vi "breaking_vigenere.vi"() -> ()   [LabVIEW 2021]
panel:
  in  "OK Button":bool
  in  "KEY":string
  out "Key Lenght":u8
  in  "freq":dbl
  out "Key":string
  out "Testo in chiaro":string
  in  "decifra":bool
  in  "Testo cifrato":string
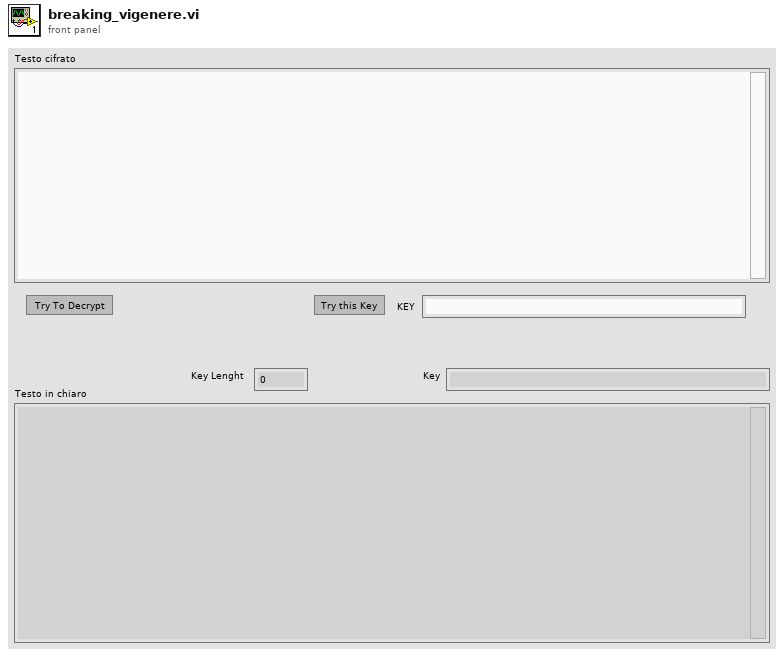
[diagram p1: front panel]
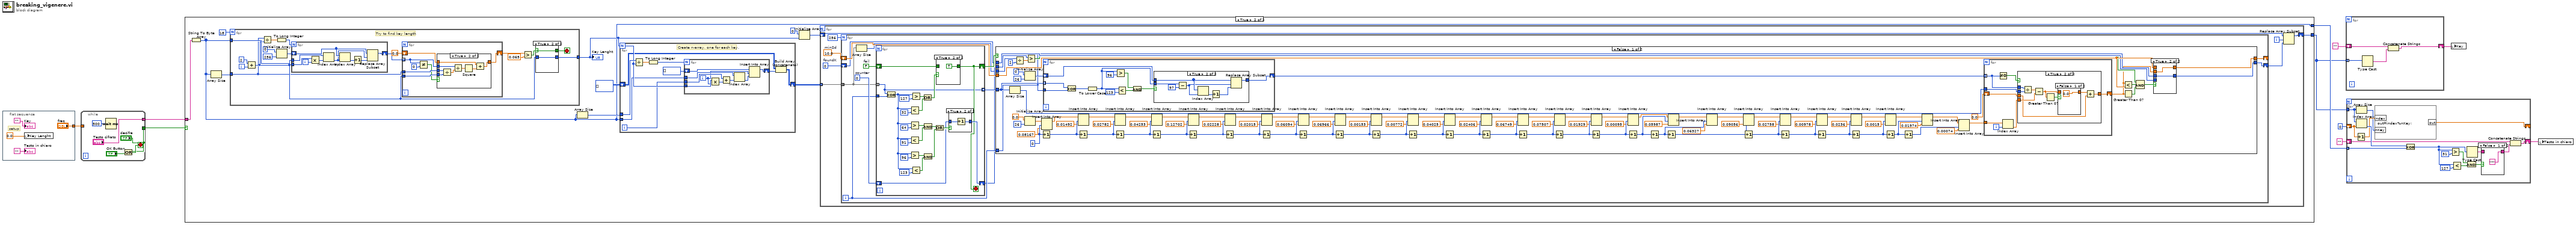
[diagram p0: block diagram]
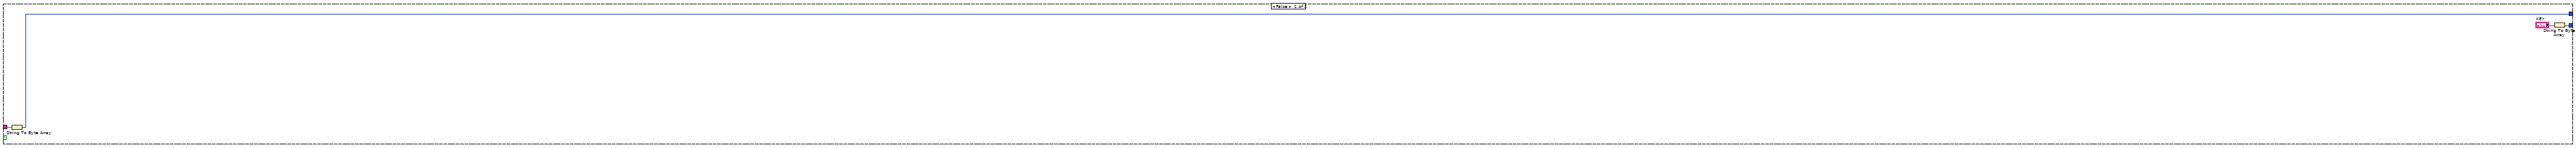
[diagram p2: hidden frame]
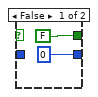
[diagram p3: hidden frame]
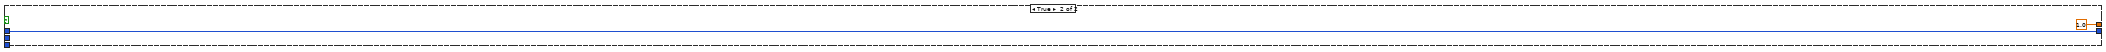
[diagram p9: hidden frame]
diagram:
  n1 = flat-sequence {
    tunnel: ["freq"] -> w5
    frame #0 {
      # "setup"
      n2 = local write "Key Lenght"(0.0 ("Key Lenght")) -> ()
      "Key" <- ""
      "Testo in chiaro" <- ""
    }
  }
  n3 = while {
    tunnel: ["Testo cifrato"] -> w10
    tunnel: w5 -> [_]
    tunnel: ["decifra"] -> w4
    stop <- w16 stop-if-true
    n4 = Wait (ms)(milliseconds to wait=u32 500) -> ()  [unwired: 1 out]
    n5 = Or(x="decifra", y="OK Button") -> (x .or. y?=w16:bool)
  }
  n6 = case shown="True" w4 {
    tunnel: w10 -> [w20 w26]
    tunnel: [w22 w30] -> w3
    tunnel: [w21 w24] -> w6
    frame False {
      n7 = String To Byte Array(string=w20) -> (unsigned byte array=w21:u8[])
      n8 = String To Byte Array(string="KEY") -> (unsigned byte array=w22:u8[])
    }
    frame True {
      n9 = String To Byte Array(string=w26) -> (unsigned byte array=w24:u8[])
      n10 = Array Size(array=w24) -> (size(s)=w28:i32)
      n11 = for {
        N: 18 -> [_]
        tunnel: w28 -> [w39]
        tunnel: w24 -> [w46]
        tunnel: [w37] -> w25
        i -> [w36]
        stop <- w35 stop-if-true
        # "Try to find key length"
        n12 = Add(x=2, y=w36) -> (x+y=w40:i32)
        n13 = Divide(x=w39, y=w40) -> (x/y=w48:dbl)
        n14 = To Long Integer(number=w48) -> (32bit integer=w47:i32)
        n15 = Initialize Array(0 ("element"), 256 ("dimension size")) -> (w45:i32[])
        n16 = for {
          N: w47 -> [_]
          tunnel: w40 -> [w79]
          tunnel: w46 -> [w78]
          shift-right: [w72] -> w44
          shift-left: w45 -> [w76]
          i -> [w80]
          n17 = Multiply(x=w79, y=w80) -> (x*y=w77:i32)
          n18 = Index Array(array=w78, index=w77) -> (element=w75:u8)
          n19 = Index Array(array=w76, index=w75) -> (element=w73:i32)
          n20 = Increment(x=w73) -> (x+1=w74:i32)
          n21 = Replace Array Subset(array=w76, new element=w74, index=w75) -> (w72:i32[])
        }
        n22 = for {
          tunnel: w44 -> [w56] mode=indexing
          tunnel: w39 -> [w62]
          tunnel: w40 -> [w61]
          shift-right: [w59] -> w42
          shift-left: 0.0 -> [w60]
          n23 = Not Equal?(x=w56, y=0) -> (x != y?=w58:bool)
          n24 = case shown="True" w58 {
            tunnel: w60 -> [w63 w71]
            tunnel: [w63 w70] -> w59
            tunnel: w62 -> [_ w69]
            tunnel: w61 -> [_ w68]
            tunnel: w56 -> [_ w64]
            frame False {
            }
            frame True {
              n25 = Divide(x=w69, y=w68) -> (x/y=w67:dbl)
              n26 = Divide(x=w64, y=w67) -> (x/y=w66:dbl)
              n27 = Square(x=w66) -> (x^2=w65:dbl)
              n28 = Add(x=w71, y=w65) -> (x+y=w70:dbl)
            }
          }
        }
        n29 = Greater?(x=w42, y=0.065) -> (0:w43:bool)
        n30 = case shown="True" w43 {
          selector: w43 -> [_ w55]
          tunnel: w40 -> [_ w54]
          tunnel: [0 w54] -> w37
          tunnel: [FALSE w55] -> w35
          frame False {
          }
          frame True {
          }
        }
      }
      "Key Lenght" <- w25
      n31 = Array Size(array=w24) -> (size(s)=w33:i32)
      n32 = for {
        N: w25 -> [w282]
        tunnel: w24 -> [w281]
        tunnel: w33 -> [w285]
        shift-right: [w277] -> w29
        shift-left: u8[][] [] -> [w276]
        i -> [w280]
        # "Create n-array, one for each key."
        n33 = Divide(x=w285, y=w282) -> (x/y=w284:dbl)
        n34 = To Long Integer(number=w284) -> (32bit integer=w283:i32)
        n35 = for {
          N: w283 -> [_]
          tunnel: w280 -> [w293]
          tunnel: w282 -> [w294]
          tunnel: w281 -> [w290]
          shift-right: [w286] -> w278
          shift-left: u8[] [] -> [w289]
          i -> [w288]
          n36 = Multiply(x=w294, y=w288) -> (x*y=w292:i32)
          n37 = Add(x=w293, y=w292) -> (x+y=w291:i32)
          n38 = Index Array(array=w290, index=w291) -> (element=w287:u8)
          n39 = Insert Into Array(array=w289, index=w288, new element=w287) -> (w286:u8[])
        }
        n40 = Build Array (concatenate)(w276, w278) -> (w277:u8[][])
      }
      n41 = Initialize Array(u8 0 ("element"), w25) -> (w31:u8[])
      n42 = for {
        tunnel: w29 -> [w85] mode=indexing
        shift-right: [w87] -> w30
        shift-left: w31 -> [w88]
        i -> [w81]
        w84 = 10.0  # minSd
        w83 = 0  # foundK
        n43 = for {
          N: 256 -> [_]
          tunnel: w85 -> [w90]
          shift-right: [w94] -> _
          shift-left: w84 -> [w95]
          shift-right: [w93] -> w82
          shift-left: w83 -> [w92]
          i -> [w96]
          w99 = 0  # counter
          w100 = FALSE  # fail
          n44 = Array Size(array=w90) -> (size(s)=w89:i32)
          n45 = for {
            tunnel: w90 -> [w248] mode=indexing
            tunnel: w96 -> [w270]
            shift-right: [w257] -> w91
            shift-left: w99 -> [w258]
            shift-right: [w249] -> w98
            shift-left: w100 -> [w250]
            tunnel: [w248] -> w97 mode=indexing
            stop <- w249 stop-if-true
            n46 = Exclusive Or(1:w270, 2:w248) -> (0:w256:i32)
            n47 = Less?(x=w256, y=32) -> (x < y?=w252:bool)
            n48 = Greater?(x=w256, y=64) -> (0:w267:bool)
            n49 = Less?(x=w256, y=91) -> (x < y?=w266:bool)
            n50 = Greater?(x=w256, y=96) -> (0:w263:bool)
            n51 = Greater?(x=w256, y=127) -> (0:w253:bool)
            n52 = Less?(x=w256, y=123) -> (x < y?=w262:bool)
            n53 = Or(x=w253, y=w252) -> (x .or. y?=w251:bool)
            n54 = And(x=w267, y=w266) -> (x .and. y?=w261:bool)
            n55 = And(x=w263, y=w262) -> (x .and. y?=w260:bool)
            n56 = Or(x=w261, y=w260) -> (x .or. y?=w259:bool)
            n57 = case shown="True" w251 {
              tunnel: w250 -> [w271 _]
              tunnel: [w271 TRUE] -> w249
              frame False {
              }
              frame True {
              }
            }
            n58 = case shown="True" w259 {
              tunnel: w258 -> [w273 w275]
              tunnel: [w273 w274] -> w257
              frame False {
              }
              frame True {
                n59 = Increment(x=w275) -> (x+1=w274:i32)
              }
            }
          }
          n60 = case shown="False" w98 {
            tunnel: w97 -> [w103 _]
            tunnel: w96 -> [w102 _]
            tunnel: w95 -> [w201 _]
            tunnel: [w202 1.0 ("Std Dev")] -> w94
            tunnel: [w200 w246] -> w93
            tunnel: w92 -> [w199 w246]
            tunnel: w91 -> [w195 _]
            tunnel: w89 -> [w192 _]
            frame False {
              w133 = 0 ("index")
              n61 = Array Size(array=w103) -> (size(s)=w189:i32)
              n62 = Divide(x=w192, y=u8 2) -> (x/y=w193:dbl)
              n63 = Initialize Array(u8 0 ("element"), 26 ("dimension size")) -> (w187:u8[])
              n64 = Initialize Array(0.0 ("element"), 26 ("dimension size")) -> (w186:dbl[])
              n65 = Greater?(x=w195, y=w193) -> (0:w191:bool)
              n66 = Increment(x=w133) -> (x+1=w181:i32)
              n67 = Insert Into Array(array=w186, index=w133, new element=0.08167 ("new element/subarray")) -> (w185:dbl[])
              n68 = for {
                tunnel: w103 -> [w233] mode=indexing
                tunnel: w102 -> [w232]
                shift-right: [w223] -> w188
                shift-left: w187 -> [w224]
                n69 = Exclusive Or(1:w232, 2:w233) -> (0:w231:i32)
                n70 = To Lower Case(string=w231) -> (all lower case string=w225:i32)
                n71 = Greater?(x=w225, y=u8 96) -> (0:w228:bool)
                n72 = Less?(x=w225, y=u8 123) -> (x < y?=w227:bool)
                n73 = And(x=w228, y=w227) -> (x .and. y?=w226:bool)
                n74 = case shown="True" w226 {
                  tunnel: w225 -> [_ w237]
                  tunnel: w224 -> [w234 w239]
                  tunnel: [w234 w238] -> w223
                  frame False {
                  }
                  frame True {
                    n75 = Subtract(x=w237, y=u8 97) -> (x-y=w235:i32)
                    n76 = Index Array(array=w239, index=w235) -> (element=w241:u8)
                    n77 = Increment(x=w241) -> (x+1=w240:u8)
                    n78 = Replace Array Subset(array=w239, new element=w240, index=w235) -> (w238:u8[])
                  }
                }
              }
              n79 = Increment(x=w181) -> (x+1=w180:i32)
              n80 = Insert Into Array(array=w185, index=w181, new element=0.01492 ("new element/subarray")) -> (w184:dbl[])
              n81 = Increment(x=w180) -> (x+1=w179:i32)
              n82 = Insert Into Array(array=w184, index=w180, new element=0.02782 ("new element/subarray")) -> (w183:dbl[])
              n83 = Increment(x=w179) -> (x+1=w178:i32)
              n84 = Insert Into Array(array=w183, index=w179, new element=0.04253 ("new element/subarray")) -> (w182:dbl[])
              n85 = Increment(x=w178) -> (x+1=w177:i32)
              n86 = Insert Into Array(array=w182, index=w178, new element=0.12702 ("new element/subarray")) -> (w172:dbl[])
              n87 = Increment(x=w177) -> (x+1=w176:i32)
              n88 = Insert Into Array(array=w172, index=w177, new element=0.02228 ("new element/subarray")) -> (w171:dbl[])
              n89 = Increment(x=w176) -> (x+1=w175:i32)
              n90 = Insert Into Array(array=w171, index=w176, new element=0.02015 ("new element/subarray")) -> (w170:dbl[])
              n91 = Increment(x=w175) -> (x+1=w174:i32)
              n92 = Insert Into Array(array=w170, index=w175, new element=0.06094 ("new element/subarray")) -> (w169:dbl[])
              n93 = Increment(x=w174) -> (x+1=w173:i32)
              n94 = Insert Into Array(array=w169, index=w174, new element=0.06966 ("new element/subarray")) -> (w168:dbl[])
              n95 = Increment(x=w173) -> (x+1=w166:i32)
              n96 = Insert Into Array(array=w168, index=w173, new element=0.00153 ("new element/subarray")) -> (w167:dbl[])
              n97 = Increment(x=w166) -> (x+1=w165:i32)
              n98 = Insert Into Array(array=w167, index=w166, new element=0.00772 ("new element/subarray")) -> (w159:dbl[])
              n99 = Increment(x=w165) -> (x+1=w164:i32)
              n100 = Insert Into Array(array=w159, index=w165, new element=0.04025 ("new element/subarray")) -> (w158:dbl[])
              n101 = Increment(x=w164) -> (x+1=w163:i32)
              n102 = Insert Into Array(array=w158, index=w164, new element=0.02406 ("new element/subarray")) -> (w157:dbl[])
              n103 = Increment(x=w163) -> (x+1=w162:i32)
              n104 = Insert Into Array(array=w157, index=w163, new element=0.06749 ("new element/subarray")) -> (w156:dbl[])
              n105 = Increment(x=w162) -> (x+1=w161:i32)
              n106 = Insert Into Array(array=w156, index=w162, new element=0.07507 ("new element/subarray")) -> (w155:dbl[])
              n107 = Increment(x=w161) -> (x+1=w160:i32)
              n108 = Insert Into Array(array=w155, index=w161, new element=0.01929 ("new element/subarray")) -> (w154:dbl[])
              n109 = Insert Into Array(array=w154, index=w160, new element=0.00095 ("new element/subarray")) -> (w153:dbl[])
              n110 = Increment(x=w160) -> (x+1=w152:i32)
              n111 = Increment(x=w152) -> (x+1=w151:i32)
              n112 = Increment(x=w151) -> (x+1=w150:i32)
              n113 = Insert Into Array(array=w153, index=w152, new element=0.05987 ("new element/subarray")) -> (w147:dbl[])
              n114 = Insert Into Array(array=w147, index=w151, new element=0.06327 ("new element/subarray")) -> (w146:dbl[])
              n115 = Increment(x=w150) -> (x+1=w149:i32)
              n116 = Insert Into Array(array=w146, index=w150, new element=0.09056 ("new element/subarray")) -> (w145:dbl[])
              n117 = Increment(x=w149) -> (x+1=w148:i32)
              n118 = Insert Into Array(array=w145, index=w149, new element=0.02758 ("new element/subarray")) -> (w144:dbl[])
              n119 = Increment(x=w148) -> (x+1=w139:i32)
              n120 = Insert Into Array(array=w144, index=w148, new element=0.00978 ("new element/subarray")) -> (w143:dbl[])
              n121 = Increment(x=w139) -> (x+1=w138:i32)
              n122 = Insert Into Array(array=w143, index=w139, new element=0.0236 ("new element/subarray")) -> (w142:dbl[])
              n123 = Insert Into Array(array=w142, index=w138, new element=0.0015 ("new element/subarray")) -> (w141:dbl[])
              n124 = Increment(x=w138) -> (x+1=w137:i32)
              n125 = Increment(x=w137) -> (x+1=w136:i32)
              n126 = Insert Into Array(array=w141, index=w137, new element=0.01974 ("new element/subarray")) -> (w140:dbl[])
              n127 = Insert Into Array(array=w140, index=w136, new element=0.00074 ("new element/subarray")) -> (w190:dbl[])
              n128 = for {
                tunnel: w188 -> [w208] mode=indexing
                shift-right: [w203] -> w101
                shift-left: 0.0 -> [w209]
                tunnel: w189 -> [w207]
                tunnel: w190 -> [w206]
                i -> [w205]
                n129 = Not Equal To 0?(x=w208) -> (x != 0?=w210:bool)
                n130 = Index Array(array=w206, index=w205) -> (element=w204:dbl)
                n131 = case shown="True" w210 {
                  tunnel: w209 -> [w211 w215]
                  tunnel: w208 -> [_ w220]
                  tunnel: w207 -> [_ w219]
                  tunnel: w204 -> [_ w217]
                  tunnel: [w211 w216] -> w203
                  frame False {
                  }
                  frame True {
                    n132 = Divide(x=w220, y=w219) -> (x/y=w218:dbl)
                    n133 = Subtract(x=w218, y=w217) -> (x-y=w213:dbl)
                    n134 = Greater Than 0?(x=w213) -> (x > 0?=w214:bool)
                    n135 = case shown="False" w214 {
                      tunnel: w213 -> [_ w222]
                      tunnel: [0.0 w222] -> w212
                      frame False {
                      }
                      frame True {
                      }
                    }
                    n136 = Add(x=w212, y=w215) -> (x+y=w216:dbl)
                  }
                }
              }
              n137 = Less?(x=w101, y=w201) -> (x < y?=w197:bool)
              n138 = Greater Than 0?(x=w101) -> (x > 0?=w196:bool)
              n139 = Compound Arithmetic op=AND(w191, w197, w196) -> (w198:bool)
              n140 = case shown="True" w198 {
                tunnel: [w243 w245] -> w202
                tunnel: w101 -> [_ w245]
                tunnel: w201 -> [w243 _]
                tunnel: [w242 w244] -> w200
                tunnel: w102 -> [_ w244]
                tunnel: w199 -> [w242 _]
                frame False {
                }
                frame True {
                }
              }
            }
            frame True {
            }
          }
        }
        n141 = Replace Array Subset(array=w88, new element=w82, index=w81) -> (w87:u8[])
      }
    }
  }
  n142 = for {
    tunnel: w3 -> [w297] mode=indexing
    shift-right: [w298] -> w2
    shift-left: "" -> [w296]
    n143 = Type Cast(x=w297) -> (*(type *) &x=w295:string)  [unwired: 1 in]
    n144 = Concatenate Strings(w296, w295) -> (w298:string)
  }
  n145 = for {
    tunnel: w6 -> [w315] mode=indexing
    tunnel: w3 -> [w308]
    shift-right: [w307] -> _
    shift-left: 0 -> [w310]
    shift-right: [w312] -> w8
    shift-left: "" -> [w313]
    n146 = Increment(x=w310) -> (x+1=w311:dbl)
    n147 = Array Size(array=w308) -> (size(s)=w309:i32)
    n148 = Index Array(array=w308, index=w310) -> (element=w314:u8)
    n149 = formula code="out=index%nKey;"("index"=w311, "nKey"=w309) -> ("out"=w307:dbl)
    n150 = Exclusive Or(1:w315, 2:w314) -> (0:w306:u8)
    n151 = Greater?(x=w306, y=u8 31) -> (0:w303:bool)
    n152 = Less?(x=w306, y=u8 127) -> (x < y?=w302:bool)
    n153 = And(x=w303, y=w302) -> (x .and. y?=w301:bool)
    n154 = Type Cast(x=w306) -> (*(type *) &x=w299:string)  [unwired: 1 in]
    n155 = case shown="False" w301 {
      tunnel: ["*" w317] -> w300
      tunnel: w299 -> [_ w317]
      frame False {
      }
      frame True {
      }
    }
    n156 = Concatenate Strings(w313, w300) -> (w312:string)
  }
  n157 = local write "Key"(w2) -> ()
  n158 = local write "Testo in chiaro"(w8) -> ()
